vi "start.vi"(8 "error in (no error)":errorcluster, 11 "DIO64Output in":refnum<class "DIO64Output.lvclass">) -> (0 "error out":errorcluster, 3 "DIO64Output out":refnum<class "DIO64Output.lvclass">)   [LabVIEW 2011, in "Hardware.lvlib" / "Channels.lvlib" / "DIO64Output.lvclass"]
uses:
  DIO64Output.lvclass
  DIO64Output.lvclass/DIO64Output.ctl
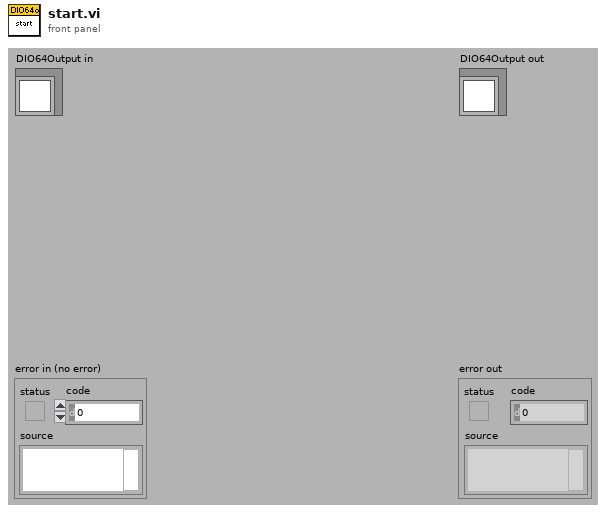
[diagram p1: front panel]
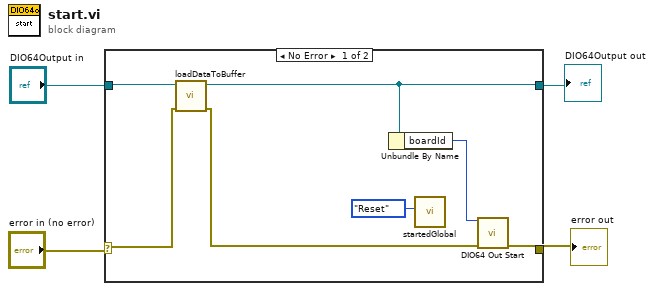
[diagram p0: block diagram]
diagram:
  n1 = case shown="No Error" "error in (no error)" {
    selector: "error in (no error)" -> [w6 w13]
    tunnel: [w11 w13] -> w3
    tunnel: "DIO64Output in" -> [w8 w12]
    tunnel: [w7 w12] -> w1
    frame No Error {
      n2 = call-dynamic "loadDataToBuffer.vi"("error in (no error)"=w6, "DIO64Output in"=w8) -> ("error out"=w5:errorcluster, "DIO64Output out"=w7:refnum<class "DIO64Output.lvclass">)  [unwired: 8 in]
      n3 = Unbundle By Name(w7) -> ("boardId"=w10:i32)
      n4 = call "startedGlobal.vi"("Action"=enum16{"Write", "Read", "Reset"}."Reset") -> ()  [unwired: 10 in, 1 out]
      n5 = call <userlib>:"DIO64 Out Start.vi"("board in"=w10, "error in (no error)"=w5) -> ("error out"=w11:errorcluster)  [unwired: 12 in, 1 out]
    }
    frame Error {
    }
  }
  "error out" <- w3
  "DIO64Output out" <- w1
